vi "RSZVB Get Reference.vi"(8 "error in (no error)":errorcluster {"code" format="%.0x"}, 11 "VISA session":refnum<visa-resource-name>) -> (0 "error out":errorcluster {"code" format="%.0x"}, 2 "Reference":i32, 3 "dup VISA session":refnum<visa-resource-name>)   [LabVIEW 2011]
doc: "This VI queries the source of the reference oscillator signal.\n\nRemote-control command(s):\n[SENSe<Ch>:]ROSCillator[:SOURce]?"
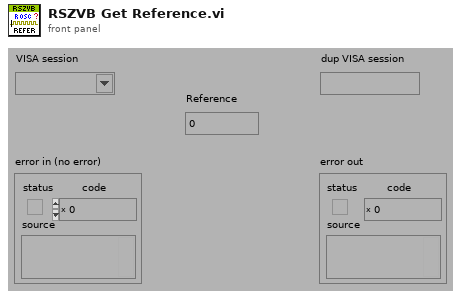
[diagram p1: front panel]
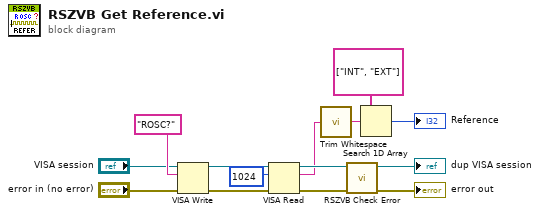
[diagram p0: block diagram]
diagram:
  n1 = VISA Write(VISA resource name="VISA session", write buffer="ROSC?", error in (no error)="error in (no error)") -> (VISA resource name out=w12:refnum<visa-resource-name>, error out=w14:errorcluster)  [unwired: 1 out]
  n2 = VISA Read(VISA resource name=w12, byte count=u32 1024 ("byte count (0)"), error in (no error)=w14) -> (VISA resource name out=w11:refnum<visa-resource-name>, read buffer=w1:string, error out=w10:errorcluster)  [unwired: 1 out]
  n3 = call <vilib>:"Trim Whitespace.vi"("string"=w1) -> ("trimmed string"=w2:string)  [unwired: 1 in]
  n4 = call "RSZVB Check Error.vi"("error in (no error)"=w10, "VISA session"=w11) -> ("error out"=→"error out":errorcluster, "dup VISA session"=→"dup VISA session":refnum<visa-resource-name>)  [unwired: 8 in]
  n5 = Search 1D Array(1D array=string[] ["INT", "EXT"] ("array 2"), element=w2) -> (index of element=→"Reference":i32)  [unwired: 1 in]
